vi "Control Panel.vi"(8 "error in (no error)":errorcluster, 11 "fake Laser Power Controller in":refnum<class "Laser Power Controller.lvclass">) -> (0 "error out":errorcluster, 3 "fake Laser Power Controller out":refnum<class "Laser Power Controller.lvclass">)   [LabVIEW 2009, in "Laser Power Controller.lvclass"]
doc: "(Dynamic) A user-level application that simulates the physical front panel of the Instrument. Provide the user with buttons to manually control features of the instrument, and provide indicators of its current state."
uses:
  Laser Power Controller.lvclass
  Utility Classes/Scannable/Scannable.lvclass
  Power Meter/Power Meter.lvclass
  Laser Power Controller.lvclass/Laser Power Controller.ctl
  BEOC LPC/BEOC LPC.lvlib
panel:
  in  "Stop Reading":bool
  out "power 2":dbl[unit] format="%.2g"
  in  "Continuous Read":bool
  out "transmission (%)":dbl format="%.2g"
  in  "transmission (%)":dbl=75.0 format="%.2g"
  in  "Set Transmission":bool
  in  "Set front-panel controls":bool
  in  "Set Control Mode":bool
  in  "Set Wavelength":bool
  in  "Set Power":bool
  out "Current Power":string
  in  "Read Power":bool
  in  "Go to Desired Power":bool
  in  "Desired Power":dbl[unit]
  in  "Configure Power Meter":bool
  in  "Read to Control":bool
  in  "Read":bool
  in  "Copy actual to set":bool
  in  "Populate fields with member data":bool
  out "front-panel controls":enum16{"enabled", "disabled"}(ring)
  out "control mode":T1(ring)
  out "wavelength":dbl[unit]
  out "power":dbl[unit] format="%.2g"
  in  "front-panel controls":enum16{"enabled", "disabled"}(ring)
  in  "control mode":T1(ring)
  in  "wavelength":dbl[unit]=8.300000000000001e-07
  in  "power":dbl[unit]=0.005 format="%.2g"
  in  "stop":bool
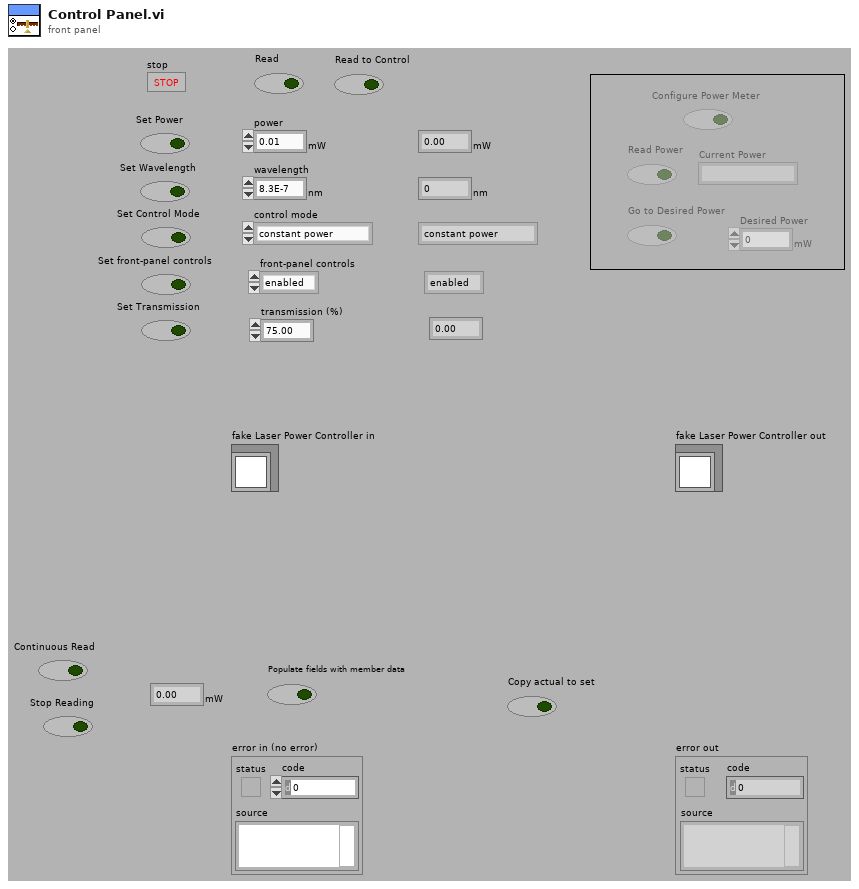
[diagram p1: front panel]
types:
  T1 = enum16{"constant power", "constant transmission"}
  T2 = enum8{"Enabled", "Disabled", "Disabled and Grayed Out"}
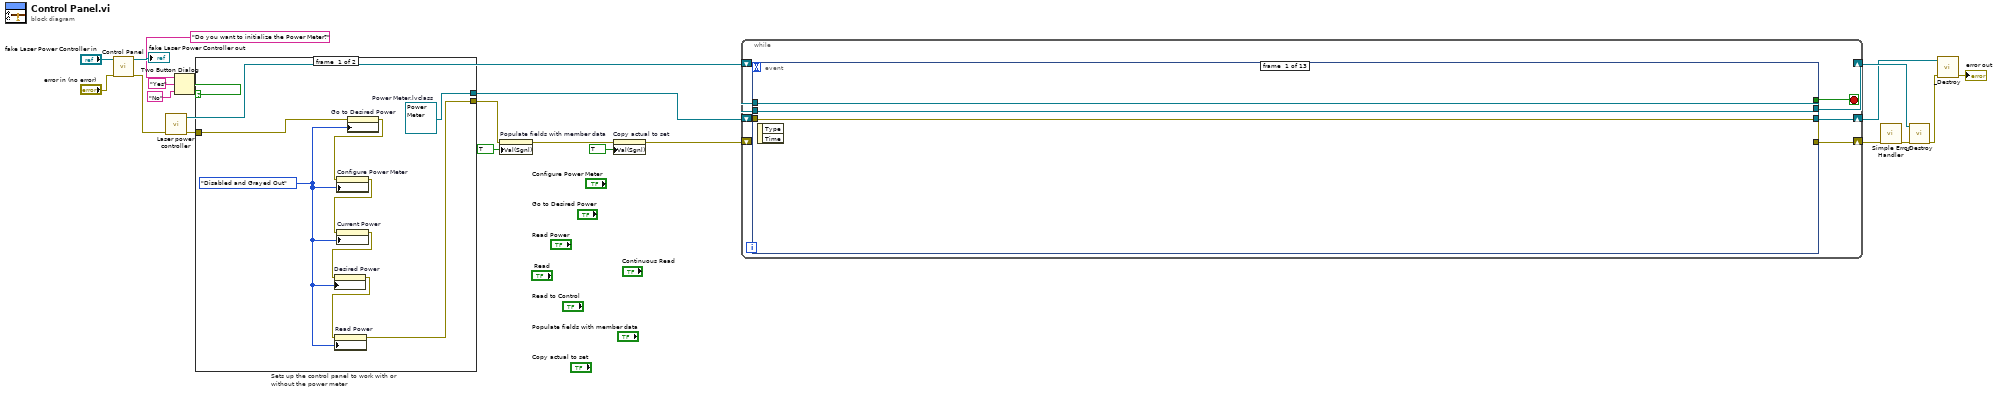
[diagram p0: block diagram]
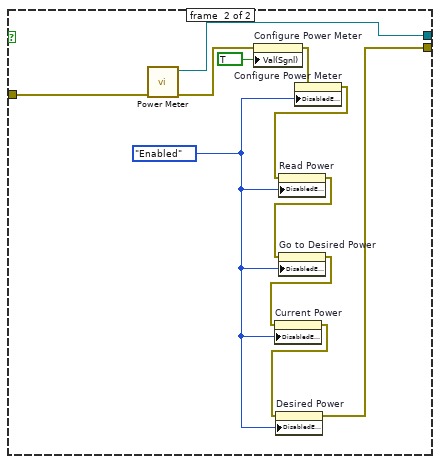
[diagram p2: hidden frame]
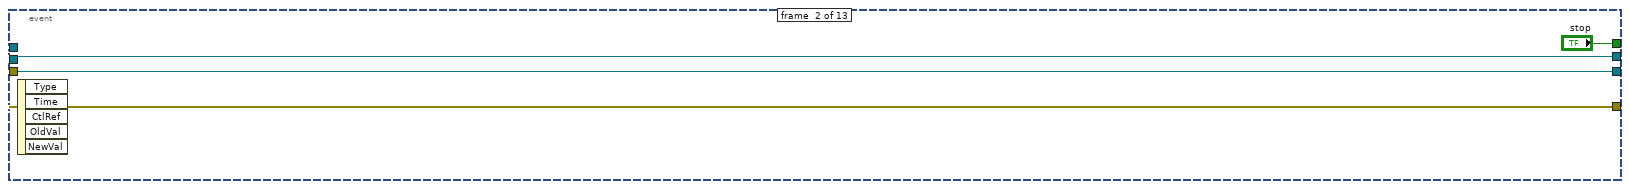
[diagram p3: hidden frame]
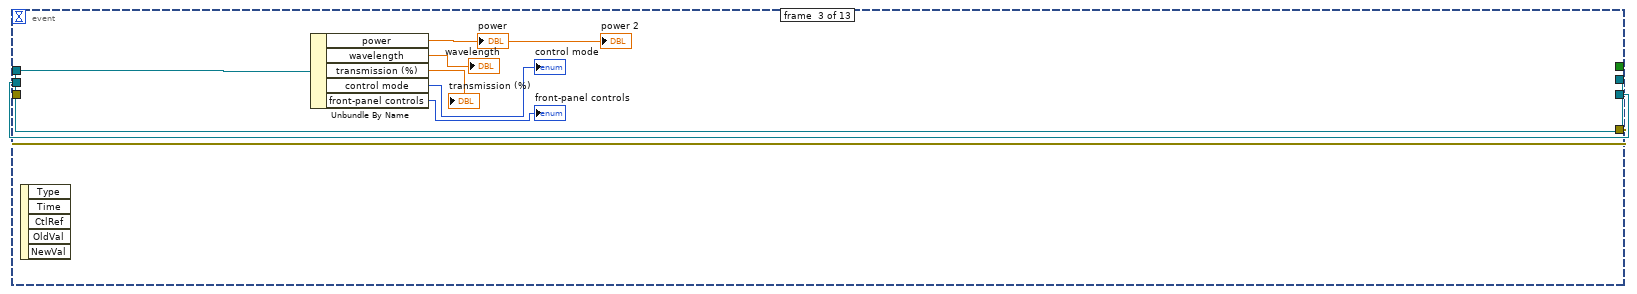
[diagram p4: hidden frame]
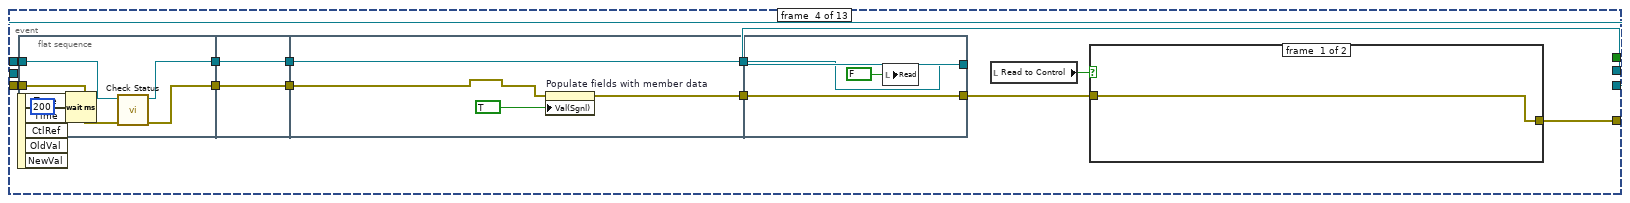
[diagram p5: hidden frame]
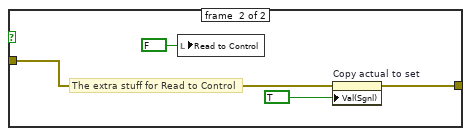
[diagram p6: hidden frame]
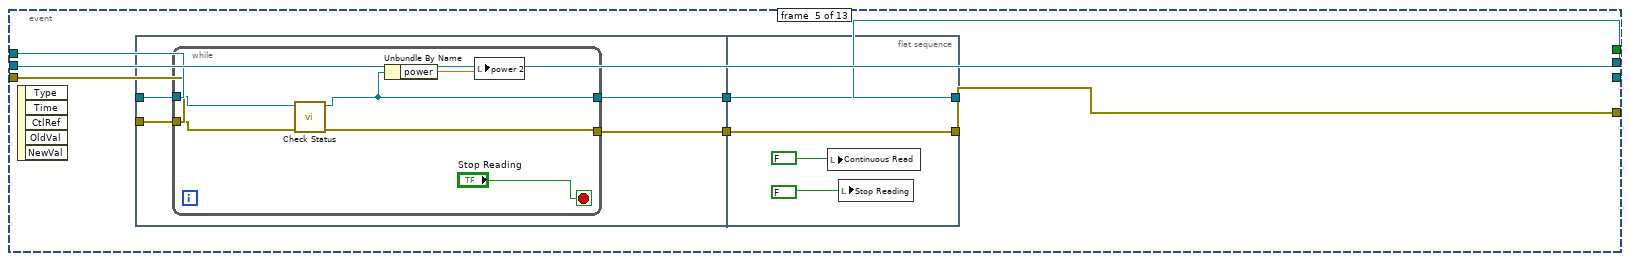
[diagram p7: hidden frame]
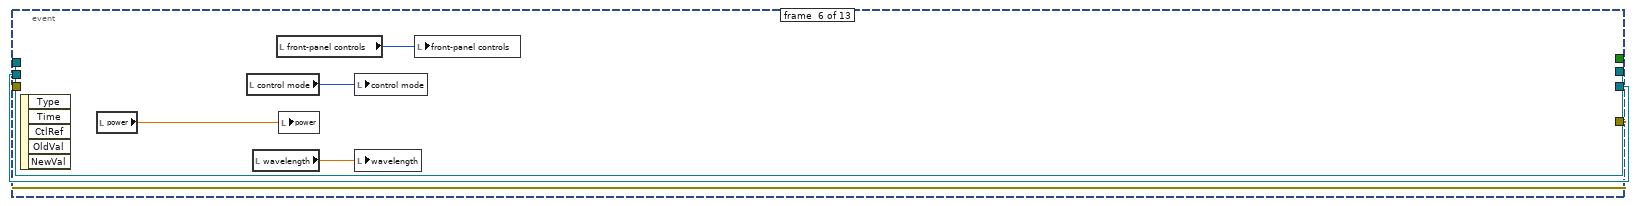
[diagram p8: hidden frame]
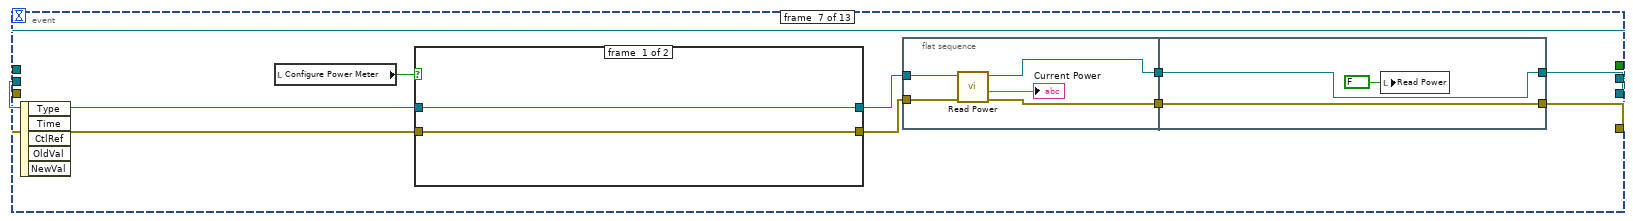
[diagram p9: hidden frame]
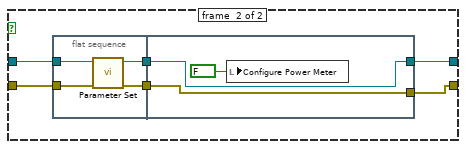
[diagram p10: hidden frame]
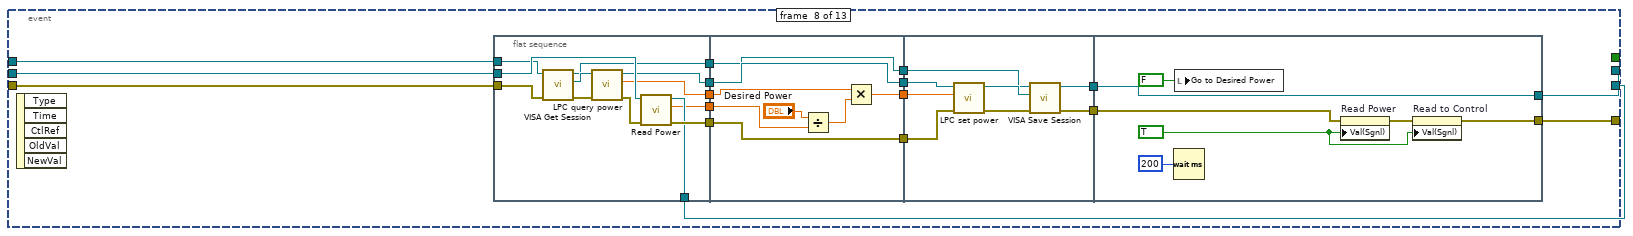
[diagram p11: hidden frame]
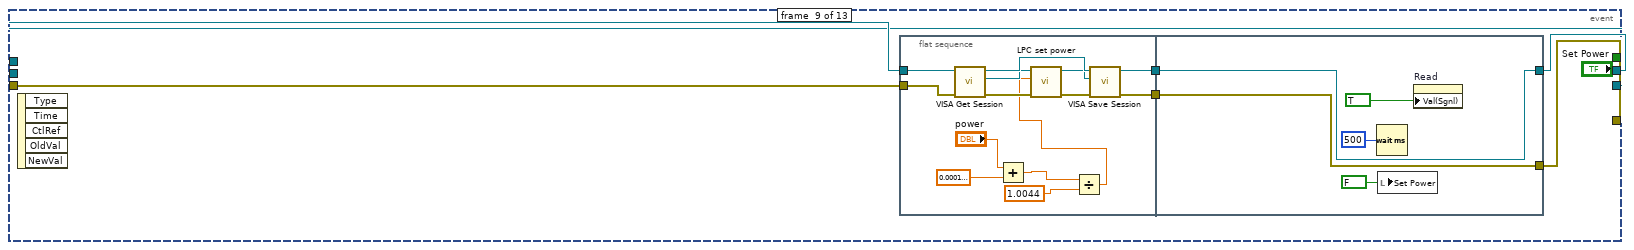
[diagram p12: hidden frame]
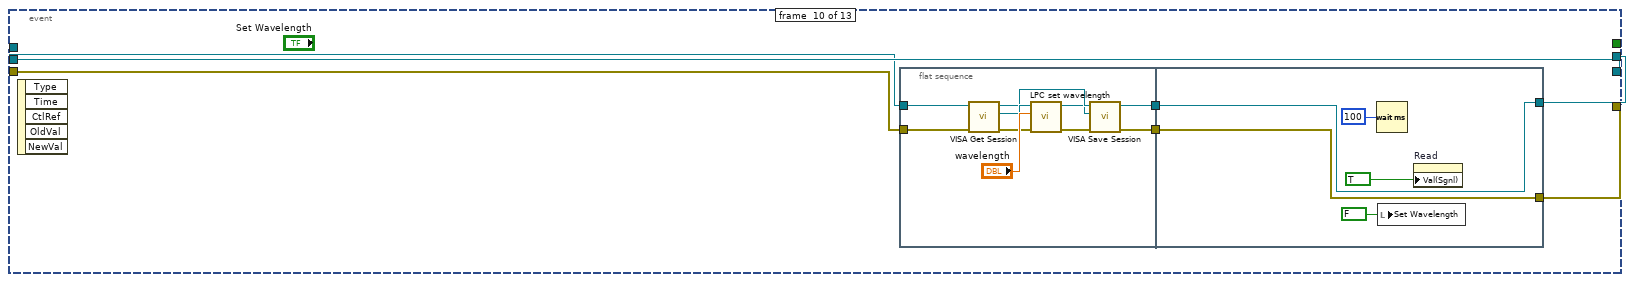
[diagram p13: hidden frame]
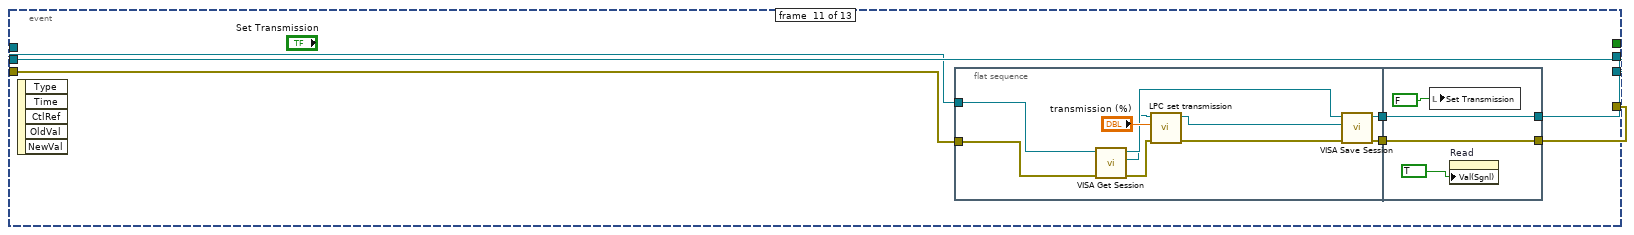
[diagram p14: hidden frame]
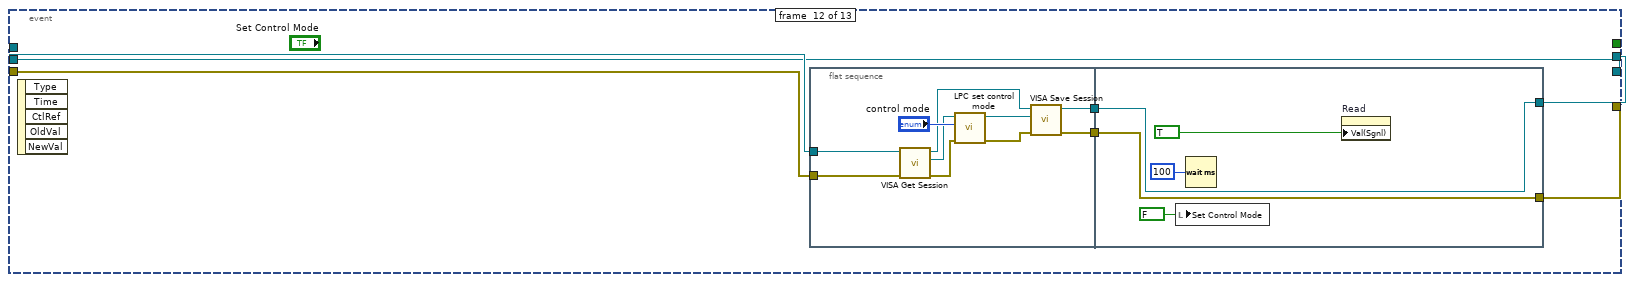
[diagram p15: hidden frame]
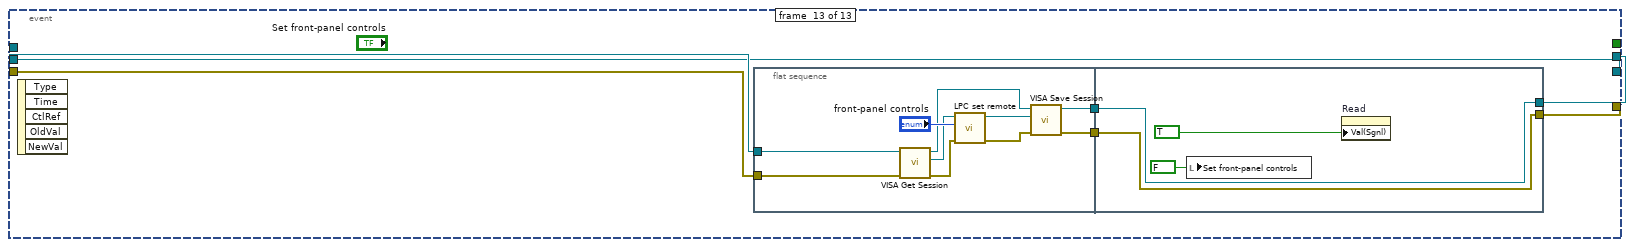
[diagram p16: hidden frame]
diagram:
  n1 = call-parent "Control Panel.vi"("error in (no error)"="error in (no error)", "Instrument in"="fake Laser Power Controller in") -> ("error out"=w19:errorcluster, "Instrument out"=→"fake Laser Power Controller out":refnum<class "Laser Power Controller.lvclass">)  [unwired: 8 in]
  n2 = call "Laser power controller.vi"("error in (no error)"=w19) -> ("error out"=w11:errorcluster, "Laser Power Controller out"=w16:refnum<class "Laser Power Controller.lvclass">)  [unwired: 9 in]
  n3 = Two Button Dialog(message="Do you want to initialize the Power Meter?", 1:"No" ("F button name (\"Cancel\")"), 2:"Yes" ("T button name (\"OK\")")) -> (T button?=w5:bool)
  n4 = case "Sets up the control panel to work with or without the power meter" shown="True" w5 {
    tunnel: w11 -> [w25 w41]
    tunnel: [w23 w31] -> w10
    tunnel: [w30 w40] -> w9
    frame #0 {
      w26 = T2."Disabled and Grayed Out" ("Disabled")
      w30 = refnum<class "Power Meter.lvclass"> refnum  # Power Meter.lvclass
      n5 = property on="Go to Desired Power" class="Bool (strict)"(error in=w25, "DisabledEnum"=w26) -> (error out=w24:errorcluster)  [unwired: 1 in, 1 out]
      n6 = property on="Configure Power Meter" class="Bool (strict)"(error in=w24, "DisabledEnum"=w26) -> (error out=w29:errorcluster)  [unwired: 1 in, 1 out]
      n7 = property on="Current Power" class="Str"(error in=w29, "DisabledEnum"=w26) -> (error out=w28:errorcluster)  [unwired: 1 in, 1 out]
      n8 = property on="Desired Power" class="DigNum (strict)"(error in=w28, "DisabledEnum"=w26) -> (error out=w27:errorcluster)  [unwired: 1 in, 1 out]
      n9 = property on="Read Power" class="Bool (strict)"(error in=w27, "DisabledEnum"=w26) -> (error out=w23:errorcluster)  [unwired: 1 in, 1 out]
    }
    frame #1 {
      w37 = T2."Enabled" ("Disabled")
      n10 = call "Power Meter.vi"("error in (no error)"=w41) -> ("error out"=w38:errorcluster, "Power Meter out"=w40:refnum<class "Power Meter.lvclass">)  [unwired: 9 in]
      n11 = property on="Configure Power Meter" class="Bool (strict)"(error in=w38, "Val(Sgnl)"=TRUE ("Value (Signaling)")) -> (error out=w36:errorcluster)  [unwired: 1 in, 1 out]
      n12 = property on="Configure Power Meter" class="Bool (strict)"(error in=w36, "DisabledEnum"=w37) -> (error out=w35:errorcluster)  [unwired: 1 in, 1 out]
      n13 = property on="Read Power" class="Bool (strict)"(error in=w35, "DisabledEnum"=w37) -> (error out=w34:errorcluster)  [unwired: 1 in, 1 out]
      n14 = property on="Go to Desired Power" class="Bool (strict)"(error in=w34, "DisabledEnum"=w37) -> (error out=w33:errorcluster)  [unwired: 1 in, 1 out]
      n15 = property on="Current Power" class="Str"(error in=w33, "DisabledEnum"=w37) -> (error out=w32:errorcluster)  [unwired: 1 in, 1 out]
      n16 = property on="Desired Power" class="DigNum (strict)"(error in=w32, "DisabledEnum"=w37) -> (error out=w31:errorcluster)  [unwired: 1 in, 1 out]
    }
  }
  n17 = property on="Populate fields with member data" class="Bool (strict)"(error in=w10, "Val(Sgnl)"=TRUE ("Value (Signaling)")) -> (error out=w18:errorcluster)  [unwired: 1 in, 1 out]
  n18 = property on="Copy actual to set" class="Bool (strict)"(error in=w18, "Val(Sgnl)"=TRUE ("Value (Signaling)")) -> (error out=w14:errorcluster)  [unwired: 1 in, 1 out]
  n19 = while {
    shift-right: [w45] -> w13
    shift-left: w16 -> [w47]
    shift-right: [w44] -> w12
    shift-left: w14 -> [w46]
    shift-right: [w42] -> w6
    shift-left: w9 -> [w43]
    stop <- w48 stop-if-true
    n20 = event shown="[7] \"Go to Desired Power\": Value Change" {
      selector: _ -> [_ _ _ _ _ _ _ _ _ _ _ _ _]
      dyn-events: _ -> [_ _ _ _ _ _ _ _ _ _ _ _ _]
      timeout: _ -> [_ _ _ _ _ _ _ _ _ _ _ _ _]
      tunnel: [_ "stop" _ _ _ _ _ _ _ _ _ _ _] -> w48
      tunnel: w47 -> [w50 w54 w62 w76 w101 w122 w133 w172 w215 w240 w262 w284 w306]
      tunnel: [w50 w54 w62 w75 w99 w122 w133 w161 w210 w235 w257 w280 w300] -> w45
      tunnel: w46 -> [w51 w53 w63 w72 w100 w123 w125 w171 w214 w239 w261 w283 w305]
      tunnel: [w51 w53 w63 w69 w98 w123 w126 w160 w209 w236 w259 w279 w302] -> w44
      tunnel: w43 -> [w49 w52 w59 w68 w102 w117 w124 w173 w213 w241 w263 w278 w304]
      tunnel: [w49 w52 w59 w68 w102 w117 w127 w159 w213 w241 w263 w278 w304] -> w42
      event #0 {
        n21 = event-data() -> ()  [unwired: 1 in, 2 out]
      }
      event #1 {
        n22 = event-data() -> ()  [unwired: 1 in, 5 out]
      }
      event #2 {
        n23 = event-data() -> ()  [unwired: 1 in, 5 out]
        n24 = Unbundle By Name(w62) -> ("power"=→"power" →"power 2":dbl[unit], "wavelength"=→"wavelength":dbl[unit], "transmission (%)"=→"transmission (%)":dbl, "control mode"=→"control mode":T1, "front-panel controls"=→"front-panel controls":enum16{"enabled", "disabled"})
      }
      event #3 {
        n25 = event-data() -> ()  [unwired: 1 in, 5 out]
        n26 = flat-sequence {
          tunnel: w72 -> [w84]
          tunnel: w76 -> [w86]
          tunnel: [w85] -> w67
          tunnel: [w83] -> w65
          tunnel: w67 -> [w88]
          tunnel: [w88] -> w66
          tunnel: w65 -> [w87]
          tunnel: [w87] -> w64
          tunnel: [w90] -> w74
          tunnel: [w91] -> w70
          tunnel: w66 -> [w90]
          tunnel: w64 -> [w89]
          tunnel: [w95] -> w75
          tunnel: w74 -> [w95]
          tunnel: [w93] -> w71
          tunnel: w70 -> [w93]
          frame #0 {
            n27 = Wait (ms)(milliseconds to wait=u32 200) -> ()  [unwired: 1 out]
            n28 = call-dynamic "Check Status.vi"("error in (no error)"=w84, "Laser Power Controller in"=w86) -> ("error out"=w83:errorcluster, "Laser Power Controller out"=w85:refnum<class "Laser Power Controller.lvclass">)  [unwired: 6 in, 2 out]
          }
          frame #1 {
          }
          frame #2 {
            n29 = property on="Populate fields with member data" class="Bool (strict)"(error in=w89, "Val(Sgnl)"=TRUE ("Value (Signaling)")) -> (error out=w91:errorcluster)  [unwired: 1 in, 1 out]
          }
          frame #3 {
            n30 = local write "Read"(FALSE ("Read")) -> ()
          }
        }
        n31 = local read "Read to Control"() -> (w73:bool)
        n32 = case shown="False" w73 {
          tunnel: w71 -> [w77 w79]
          tunnel: [w77 w78] -> w69
          frame #0 {
          }
          frame #1 {
            # "The extra stuff for Read to Control"
            n33 = local write "Read to Control"(FALSE ("Read to Control")) -> ()
            n34 = property on="Copy actual to set" class="Bool (strict)"(error in=w79, "Val(Sgnl)"=TRUE ("Value (Signaling)")) -> (error out=w78:errorcluster)  [unwired: 1 in, 1 out]
          }
        }
      }
      event #4 {
        n35 = event-data() -> ()  [unwired: 1 in, 5 out]
        n36 = flat-sequence {
          tunnel: w101 -> [w106]
          tunnel: w100 -> [w105]
          tunnel: [w104] -> w97
          tunnel: [w103] -> w96
          tunnel: [w115] -> w98
          tunnel: [w116] -> w99
          tunnel: w97 -> [w116]
          tunnel: w96 -> [w115]
          frame #0 {
            n37 = while {
              tunnel: w106 -> [w112]
              tunnel: w105 -> [w111]
              tunnel: [w109] -> w104
              tunnel: [w110] -> w103
              stop <- "Stop Reading" stop-if-true
              n38 = call-dynamic "Check Status.vi"("error in (no error)"=w111, "Laser Power Controller in"=w112) -> ("error out"=w110:errorcluster, "Laser Power Controller out"=w109:refnum<class "Laser Power Controller.lvclass">)  [unwired: 6 in, 2 out]
              n39 = Unbundle By Name(w109) -> ("power"=w108:dbl[unit])
              n40 = local write "power 2"(w108) -> ()
            }
          }
          frame #1 {
            n41 = local write "Continuous Read"(FALSE) -> ()
            n42 = local write "Stop Reading"(FALSE) -> ()
          }
        }
      }
      event #5 {
        n43 = event-data() -> ()  [unwired: 1 in, 5 out]
        n44 = local read "power"() -> (w121:dbl[unit])
        n45 = local read "control mode"() -> (w119:T1)
        n46 = local read "wavelength"() -> (w120:dbl[unit])
        n47 = local read "front-panel controls"() -> (w118:enum16{"enabled", "disabled"})
        n48 = local write "power"(w121) -> ()
        n49 = local write "control mode"(w119) -> ()
        n50 = local write "wavelength"(w120) -> ()
        n51 = local write "front-panel controls"(w118) -> ()
      }
      event #6 {
        n52 = event-data() -> ()  [unwired: 1 in, 5 out]
        n53 = local read "Configure Power Meter"() -> (w132:bool)
        n54 = case shown="True" w132 {
          tunnel: w125 -> [w142 w149]
          tunnel: w124 -> [w143 w148]
          tunnel: [w143 w146] -> w128
          tunnel: [w142 w144] -> w129
          frame #0 {
          }
          frame #1 {
            n55 = flat-sequence {
              tunnel: w149 -> [w153]
              tunnel: w148 -> [w152]
              tunnel: [w151] -> w147
              tunnel: [w150] -> w145
              tunnel: w147 -> [w155]
              tunnel: [w155] -> w146
              tunnel: w145 -> [w154]
              tunnel: [w154] -> w144
              frame #0 {
                n56 = call "Parameter Set.vi"("error in (no error)"=w153, "Power Meter in"=w152) -> ("error out"=w150:errorcluster, "Power Meter out"=w151:refnum<class "Power Meter.lvclass">)  [unwired: 8 in]
              }
              frame #1 {
                n57 = local write "Configure Power Meter"(FALSE ("Value (Signaling)")) -> ()
              }
            }
          }
        }
        n58 = flat-sequence {
          tunnel: [w136] -> w131
          tunnel: [w135] -> w130
          tunnel: w128 -> [w138]
          tunnel: w129 -> [w137]
          tunnel: [w141] -> w127
          tunnel: [w139] -> w126
          tunnel: w131 -> [w139]
          tunnel: w130 -> [w141]
          frame #0 {
            n59 = call "Read Power.vi"("error in (no error)"=w137, "Power Meter in"=w138) -> ("error out"=w136:errorcluster, "Current Power w/ Units"=→"Current Power":string, "Power Meter out"=w135:refnum<class "Power Meter.lvclass">)  [unwired: 6 in, 1 out]
          }
          frame #1 {
            n60 = local write "Read Power"(FALSE ("Value (Signaling)")) -> ()
          }
        }
      }
      event #7 {
        n61 = event-data() -> ()  [unwired: 1 in, 5 out]
        n62 = flat-sequence {
          tunnel: w173 -> [w185]
          tunnel: w172 -> [w184]
          tunnel: w171 -> [w183]
          tunnel: [w179] -> w169
          tunnel: [w178] -> w168
          tunnel: [w174] -> w167
          tunnel: [w177] -> w164
          tunnel: [w176] -> w162
          tunnel: [w175] -> w159
          tunnel: [w193] -> w170
          tunnel: w169 -> [w193]
          tunnel: w168 -> [w188]
          tunnel: w167 -> [w189]
          tunnel: [w186] -> w166
          tunnel: [w192] -> w165
          tunnel: w164 -> [w192]
          tunnel: [w191] -> w163
          tunnel: w162 -> [w191]
          tunnel: w170 -> [w201]
          tunnel: w166 -> [w194]
          tunnel: w165 -> [w199]
          tunnel: w163 -> [w198]
          tunnel: [w196] -> w158
          tunnel: [w195] -> w157
          tunnel: [w206] -> w160
          tunnel: [w208] -> w161
          tunnel: w158 -> [w208]
          tunnel: w157 -> [w203]
          frame #0 {
            n63 = call-dynamic "VISA Get Session.vi"("error in (no error)"=w183, "Instrument.lvclass in"=w184) -> ("error out"=w181:errorcluster, "VISA Resource Name"=w182:refnum<visa-resource-name>, "Instrument.lvclass out"=w177:refnum<class "Laser Power Controller.lvclass">)  [unwired: 6 in, 1 out]
            n64 = call "LPC query power.vi"("error in (no error)"=w181, "VISA resource name"=w182) -> ("error out"=w180:errorcluster, "power"=w178:dbl[unit], "VISA resource name out"=w179:refnum<visa-resource-name>)  [unwired: 7 in]
            n65 = call "Read Power.vi"("error in (no error)"=w180, "Power Meter in"=w185) -> ("error out"=w176:errorcluster, "Current Power"=w174:dbl[unit], "Power Meter out"=w175:refnum<class "Power Meter.lvclass">)  [unwired: 6 in, 1 out]
          }
          frame #1 {
            n66 = Divide(x="Desired Power", y=w189) -> (x/y=w187:dbl)
            n67 = Multiply(x=w188, y=w187) -> (x*y=w186:dbl[unit])
          }
          frame #2 {
            n68 = call "LPC set power.vi"("error in (no error)"=w198, "power"=w194, "VISA resource name"=w201) -> ("error out"=w197:errorcluster, "VISA resource name out"=w200:refnum<visa-resource-name>)  [unwired: 7 in]
            n69 = call-dynamic "VISA Save Session.vi"("error in (no error)"=w197, "VISA Resource Name"=w200, "Instrument.lvclass in"=w199) -> ("error out"=w195:errorcluster, "Instrument.lvclass out"=w196:refnum<class "Laser Power Controller.lvclass">)  [unwired: 7 in]
          }
          frame #3 {
            w204 = TRUE ("Value (Signaling)")
            n70 = Wait (ms)(milliseconds to wait=u32 200) -> ()  [unwired: 1 out]
            n71 = local write "Go to Desired Power"(FALSE ("Go to Desired Power")) -> ()
            n72 = property on="Read Power" class="Bool (strict)"(error in=w203, "Val(Sgnl)"=w204) -> (error out=w205:errorcluster)  [unwired: 1 in, 1 out]
            n73 = property on="Read to Control" class="Bool (strict)"(error in=w205, "Val(Sgnl)"=w204) -> (error out=w206:errorcluster)  [unwired: 1 in, 1 out]
          }
        }
      }
      event #8 {
        n74 = event-data() -> ()  [unwired: 1 in, 5 out]
        n75 = flat-sequence {
          tunnel: w215 -> [w229]
          tunnel: w214 -> [w228]
          tunnel: [w222] -> w212
          tunnel: [w221] -> w211
          tunnel: w212 -> [w233]
          tunnel: w211 -> [w234]
          tunnel: [w234] -> w210
          tunnel: [w233] -> w209
          frame #0 {
            n76 = call-dynamic "VISA Get Session.vi"("error in (no error)"=w228, "Instrument.lvclass in"=w229) -> ("error out"=w227:errorcluster, "VISA Resource Name"=w223:refnum<visa-resource-name>, "Instrument.lvclass out"=w225:refnum<class "Laser Power Controller.lvclass">)  [unwired: 7 out]
            n77 = Add(x="power", y=dbl[unit] 0.00011899999999999999) -> (x+y=w219:dbl[unit])
            n78 = Divide(x=w219, y=1.0044) -> (x/y=w216:dbl[unit])
            n79 = call "LPC set power.vi"("error in (no error)"=w227, "power"=w216, "VISA resource name"=w223) -> ("error out"=w226:errorcluster, "VISA resource name out"=w224:refnum<visa-resource-name>)  [unwired: 7 in]
            n80 = call-dynamic "VISA Save Session.vi"("error in (no error)"=w226, "VISA Resource Name"=w224, "Instrument.lvclass in"=w225) -> ("error out"=w222:errorcluster, "Instrument.lvclass out"=w221:refnum<class "Laser Power Controller.lvclass">)  [unwired: 7 out]
          }
          frame #1 {
            n81 = Wait (ms)(milliseconds to wait=u32 500) -> ()  [unwired: 1 out]
            n82 = local write "Set Power"(FALSE) -> ()
            n83 = property on="Read" class="Bool (strict)"("Val(Sgnl)"=TRUE) -> ()  [unwired: 2 in, 2 out]
          }
        }
      }
      event #9 {
        n84 = event-data() -> ()  [unwired: 1 in, 5 out]
        n85 = flat-sequence {
          tunnel: w240 -> [w249]
          tunnel: w239 -> [w248]
          tunnel: [w243] -> w238
          tunnel: [w242] -> w237
          tunnel: w238 -> [w255]
          tunnel: w237 -> [w256]
          tunnel: [w256] -> w235
          tunnel: [w255] -> w236
          frame #0 {
            n86 = call-dynamic "VISA Get Session.vi"("error in (no error)"=w248, "Instrument.lvclass in"=w249) -> ("error out"=w245:errorcluster, "VISA Resource Name"=w250:refnum<visa-resource-name>, "Instrument.lvclass out"=w247:refnum<class "Laser Power Controller.lvclass">)  [unwired: 7 out]
            n87 = call "LPC set wavelength.vi"("error in (no error)"=w245, "wavelength"="wavelength", "VISA resource name"=w250) -> ("error out"=w244:errorcluster, "VISA resource name out"=w246:refnum<visa-resource-name>)  [unwired: 7 in]
            n88 = call-dynamic "VISA Save Session.vi"("error in (no error)"=w244, "VISA Resource Name"=w246, "Instrument.lvclass in"=w247) -> ("error out"=w243:errorcluster, "Instrument.lvclass out"=w242:refnum<class "Laser Power Controller.lvclass">)  [unwired: 7 out]
          }
          frame #1 {
            n89 = Wait (ms)(milliseconds to wait=u32 100) -> ()  [unwired: 1 out]
            n90 = local write "Set Wavelength"(FALSE) -> ()
            n91 = property on="Read" class="Bool (strict)"("Val(Sgnl)"=TRUE) -> ()  [unwired: 2 in, 2 out]
          }
        }
      }
      event #10 {
        n92 = event-data() -> ()  [unwired: 1 in, 5 out]
        n93 = flat-sequence {
          tunnel: w262 -> [w273]
          tunnel: w261 -> [w272]
          tunnel: [w268] -> w260
          tunnel: [w266] -> w258
          tunnel: w260 -> [w277]
          tunnel: [w277] -> w259
          tunnel: w258 -> [w276]
          tunnel: [w276] -> w257
          frame #0 {
            n94 = call-dynamic "VISA Get Session.vi"("error in (no error)"=w272, "Instrument.lvclass in"=w273) -> ("error out"=w270:errorcluster, "VISA Resource Name"=w265:refnum<visa-resource-name>, "Instrument.lvclass out"=w267:refnum<class "Laser Power Controller.lvclass">)  [unwired: 7 out]
            n95 = call "LPC set transmission.vi"("error in (no error)"=w270, "transmission (%)"="transmission (%)", "VISA resource name"=w265) -> ("error out"=w269:errorcluster, "VISA resource name out"=w264:refnum<visa-resource-name>)  [unwired: 7 in]
            n96 = call-dynamic "VISA Save Session.vi"("error in (no error)"=w269, "VISA Resource Name"=w264, "Instrument.lvclass in"=w267) -> ("error out"=w268:errorcluster, "Instrument.lvclass out"=w266:refnum<class "Laser Power Controller.lvclass">)  [unwired: 7 out]
          }
          frame #1 {
            n97 = local write "Set Transmission"(FALSE) -> ()
            n98 = property on="Read" class="Bool (strict)"("Val(Sgnl)"=TRUE) -> ()  [unwired: 2 in, 2 out]
          }
        }
      }
      event #11 {
        n99 = event-data() -> ()  [unwired: 1 in, 5 out]
        n100 = flat-sequence {
          tunnel: w284 -> [w288]
          tunnel: w283 -> [w287]
          tunnel: [w286] -> w282
          tunnel: [w285] -> w281
          tunnel: w282 -> [w298]
          tunnel: w281 -> [w299]
          tunnel: [w299] -> w279
          tunnel: [w298] -> w280
          frame #0 {
            n101 = call-dynamic "VISA Get Session.vi"("error in (no error)"=w287, "Instrument.lvclass in"=w288) -> ("error out"=w293:errorcluster, "VISA Resource Name"=w291:refnum<visa-resource-name>, "Instrument.lvclass out"=w289:refnum<class "Laser Power Controller.lvclass">)  [unwired: 7 out]
            n102 = call "LPC set control mode.vi"("error in (no error)"=w293, "control mode"="control mode", "VISA resource name"=w291) -> ("error out"=w292:errorcluster, "VISA resource name out"=w290:refnum<visa-resource-name>)  [unwired: 7 in]
            n103 = call-dynamic "VISA Save Session.vi"("error in (no error)"=w292, "VISA Resource Name"=w290, "Instrument.lvclass in"=w289) -> ("error out"=w285:errorcluster, "Instrument.lvclass out"=w286:refnum<class "Laser Power Controller.lvclass">)  [unwired: 7 out]
          }
          frame #1 {
            n104 = local write "Set Control Mode"(FALSE) -> ()
            n105 = Wait (ms)(milliseconds to wait=u32 100) -> ()  [unwired: 1 out]
            n106 = property on="Read" class="Bool (strict)"("Val(Sgnl)"=TRUE) -> ()  [unwired: 2 in, 2 out]
          }
        }
      }
      event #12 {
        n107 = event-data() -> ()  [unwired: 1 in, 5 out]
        n108 = flat-sequence {
          tunnel: w306 -> [w315]
          tunnel: w305 -> [w314]
          tunnel: [w311] -> w303
          tunnel: [w309] -> w301
          tunnel: w303 -> [w320]
          tunnel: [w320] -> w302
          tunnel: w301 -> [w319]
          tunnel: [w319] -> w300
          frame #0 {
            n109 = call-dynamic "VISA Get Session.vi"("error in (no error)"=w314, "Instrument.lvclass in"=w315) -> ("error out"=w313:errorcluster, "VISA Resource Name"=w308:refnum<visa-resource-name>, "Instrument.lvclass out"=w310:refnum<class "Laser Power Controller.lvclass">)  [unwired: 7 out]
            n110 = call "LPC set remote.vi"("error in (no error)"=w313, "front-panel controls"="front-panel controls", "VISA resource name"=w308) -> ("error out"=w312:errorcluster, "VISA resource name out"=w307:refnum<visa-resource-name>)  [unwired: 7 in]
            n111 = call-dynamic "VISA Save Session.vi"("error in (no error)"=w312, "VISA Resource Name"=w307, "Instrument.lvclass in"=w310) -> ("error out"=w311:errorcluster, "Instrument.lvclass out"=w309:refnum<class "Laser Power Controller.lvclass">)  [unwired: 7 out]
          }
          frame #1 {
            n112 = local write "Set front-panel controls"(FALSE) -> ()
            n113 = property on="Read" class="Bool (strict)"("Val(Sgnl)"=TRUE) -> ()  [unwired: 2 in, 2 out]
          }
        }
      }
    }
  }
  n114 = call <vilib>:"Simple Error Handler.vi"("error in (no error)"=w12) -> ("error out"=w15:errorcluster)  [unwired: 1 in, 7 out]
  n115 = call-dynamic "_Destroy.vi"("error in (no error)"=w15, "Instrument in"=w13) -> ("error out"=w8:errorcluster)  [unwired: 9 out]
  n116 = call-dynamic "_Destroy.vi"("error in (no error)"=w8, "Instrument in"=w6) -> ("error out"=→"error out":errorcluster)  [unwired: 9 out]
